vi "ge_CellIndicators.vi"(6 "MeasType":T3, 7 "ge_DAQManDefinitions":T1, 8 "error in":errorcluster, 9 "Cell Contents":string, 10 "ActiveCell":T2, 11 "Item Names":string[][](array[string])) -> (0 "error out":errorcluster, 3 "Item Names":string[][](array[string]))   [LabVIEW 2012]
uses:
  Custom Ctrls/ge_MeasType.ctl
  <vilib>/Utility/miscctls.llb/LVRowAndColumnTypeDef.ctl
  Common/Controls/DAQMan Definitions.ctl
  Common/Controls/HeaderNames.ctl
  Classes/Measurements/Class Channel/Channel.lvclass
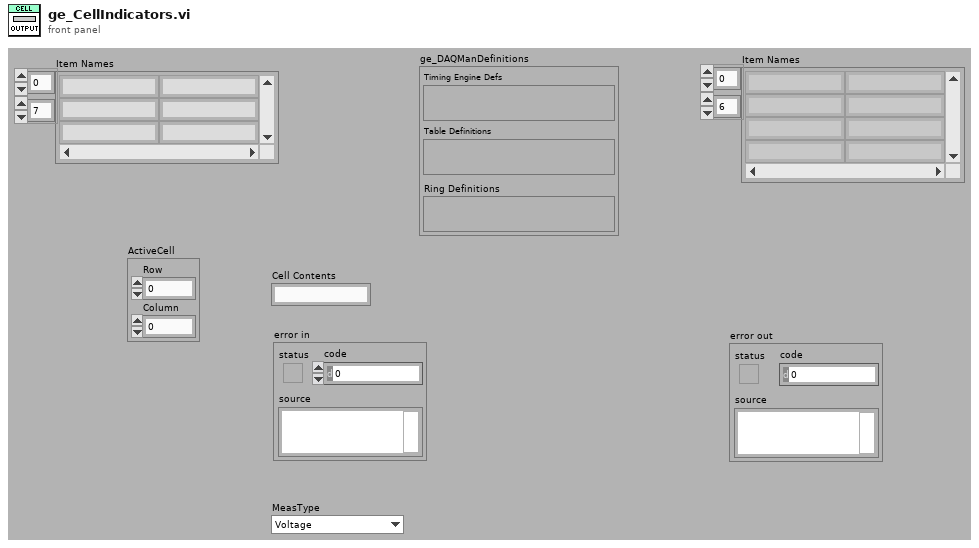
[diagram p1: front panel]
types:
  T1 = typedef "DAQMan Definitions.ctl" = cluster{"Timing Engine Defs":variant, "Table Definitions":variant, "Ring Definitions":variant}
  T2 = typedef "LVRowAndColumnTypeDef.ctl" = cluster{"Row":i32, "Column":i32}
  T3 = typedef "ge_MeasType.ctl" = enum16{"Voltage", "Frequency", "Tachometer", "Dynamic", "Thermocouple", "RTD", "Strain", "Current", "Resistance"}
  T4 = typedef "HeaderNames.ctl" = enum16{"Channel", "Device", "Spacer", "Description", "MB", "Range", "Terminal", "Coupling", "Thresh (V)", "Pulse/Rev", "Slope", "Min EU", "Min RPM", "mV/EU", "Iex", "Temp Units", "Type", "CJC Src", "CJC Val", "Ro", "Wire Cfg", "Strain Mode", "Vex", "Bridge Type", "GF", "Gauge Res", "Poisson", "Lead Res", "Init Strain", "GAF", "Scale", "Offset", "Unit (EU)", "dB?", "dB Ref", "Cal Mag", "Cal Units", "Max Temp", "Min Temp", "Max Strain", "Min Strain"}
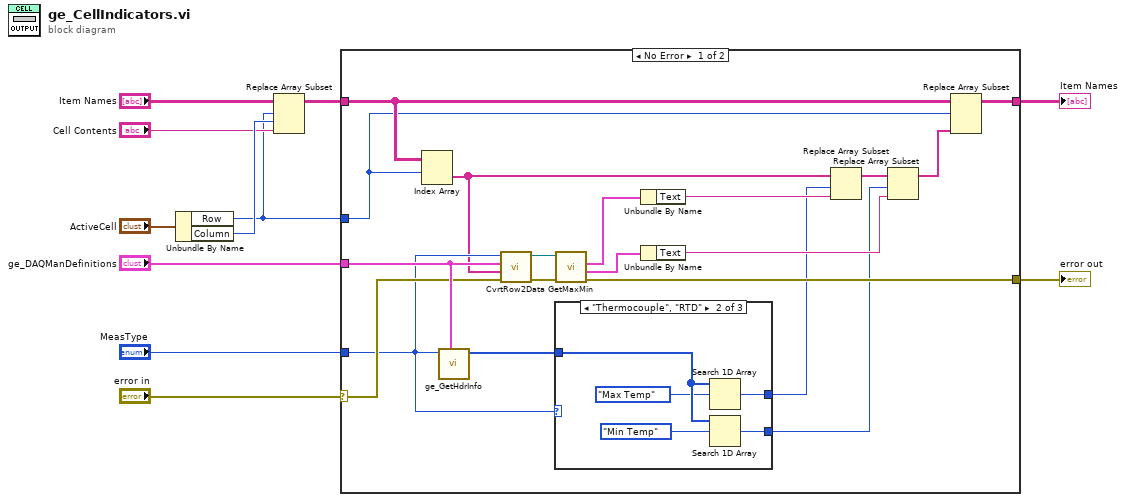
[diagram p0: block diagram]
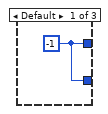
[diagram p2: hidden frame]
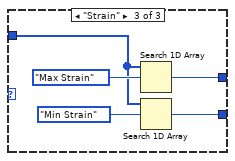
[diagram p3: hidden frame]
diagram:
  n1 = Unbundle By Name("ActiveCell") -> ("Row"=w4:i32, "Column"=w8:i32)
  n2 = Replace Array Subset(array="Item Names", new element="Cell Contents", index (row)=w4, index (col)=w8) -> (w5:string[][])
  n3 = case shown="No Error" "error in" {
    selector: "error in" -> [w25 w43]
    tunnel: [w17 w43] -> w11
    tunnel: "MeasType" -> [w13 _]
    tunnel: w5 -> [w29 w42]
    tunnel: w4 -> [w28 _]
    tunnel: [w27 w42] -> w9
    tunnel: "ge_DAQManDefinitions" -> [w26 _]
    frame No Error {
      n4 = Index Array(array=w29, index (row)=w28) -> (element=w12:string[])  [unwired: 1 in]
      n5 = call "ge_GetHdrInfo.vi"("ge_DAQManDefinitions"=w26, "MeasType"=w13) -> ("Hdr Name"=w16:T4[])  [unwired: 7 in, 2 out]
      n6 = call "CvrtRow2Data.vi"("error in (no error)"=w25, "Item Names"=w12, "ge_DAQManDefinitions"=w26, "MeasType"=w13) -> ("error out"=w23:errorcluster, "Channel out"=w24:refnum<class "Channel.lvclass">)  [unwired: 6 in]
      n7 = case shown="\"Thermocouple\", \"RTD\"" w13 {
        tunnel: w16 -> [_ w34 w39]
        tunnel: [w31 w36 w38] -> w15
        tunnel: [w31 w35 w37] -> w14
        frame Default {
          w31 = -1 ("index of element")
        }
        frame "Thermocouple", "RTD" {
          n8 = Search 1D Array(1D array=w34, element=HeaderNames."Max Temp") -> (index of element=w36:i32)  [unwired: 1 in]
          n9 = Search 1D Array(1D array=w34, element=HeaderNames."Min Temp") -> (index of element=w35:i32)  [unwired: 1 in]
        }
        frame "Strain" {
          n10 = Search 1D Array(1D array=w39, element=HeaderNames."Max Strain") -> (index of element=w38:i32)  [unwired: 1 in]
          n11 = Search 1D Array(1D array=w39, element=HeaderNames."Min Strain") -> (index of element=w37:i32)  [unwired: 1 in]
        }
      }
      n12 = call-dynamic "GetMaxMin.vi"("error in (no error)"=w23, "Channel in"=w24) -> ("error out"=w17:errorcluster, "Min"=w21:cluster{"Value":dbl, "Text":string}, "Max"=w22:cluster{"Value":dbl, "Text":string})  [unwired: 6 in, 1 out]
      n13 = Unbundle By Name(w22) -> ("Text"=w19:string)
      n14 = Unbundle By Name(w21) -> ("Text"=w18:string)
      n15 = Replace Array Subset(array=w12, new element=w19, index=w15) -> (w20:string[])
      n16 = Replace Array Subset(array=w20, new element=w18, index=w14) -> (w30:string[])
      n17 = Replace Array Subset(array=w29, new element=w30, index (row)=w28) -> (w27:string[][])  [unwired: 1 in]
    }
    frame Error {
    }
  }
  "error out" <- w11
  "Item Names" <- w9
